vi "test_CCDAcquisitionSequenceSpectrum.vi"(0 "device selection":enum16{"monochromator", "CCD", "SCD"}(ring)=enum."CCD", 1 "Test should pass":bool=TRUE, 5 "set-up a connection":bool=TRUE, 7 "set 3 ROIs / set 1 ROI":bool=TRUE, 9 "tear down connection":bool=TRUE, 11 "error in":errorcluster, 12 "activate logger?":bool, 13 "Handler Name":string="example logger handler") -> (2 "ready":bool, 3 "log-file path":path, 4 "results-JSON string":string, 6 "xyData":dbl[][][][](array[numeric]), 8 "meta data":T1[][](array[typedef]), 15 "error out":errorcluster)   [LabVIEW 2023]
uses:
  Classes/CCD/CCDSpectralData.ctl
  Classes/CCD/XAxisConversionTypeEnum.ctl
  Classes/CCD/AcquisitionFormatEnum.ctl
  Classes/CCD/CCD.lvclass
  <vilib>/addons/_JKI Toolkits/Caraya/classes/Assert/Assert Not Error.vi
  <vilib>/addons/_JKI Toolkits/Caraya/classes/Test/Test.lvclass
  <vilib>/addons/_JKI Toolkits/Caraya/classes/Assert/Assert.lvclass
panel:
  # "Connector Pane"
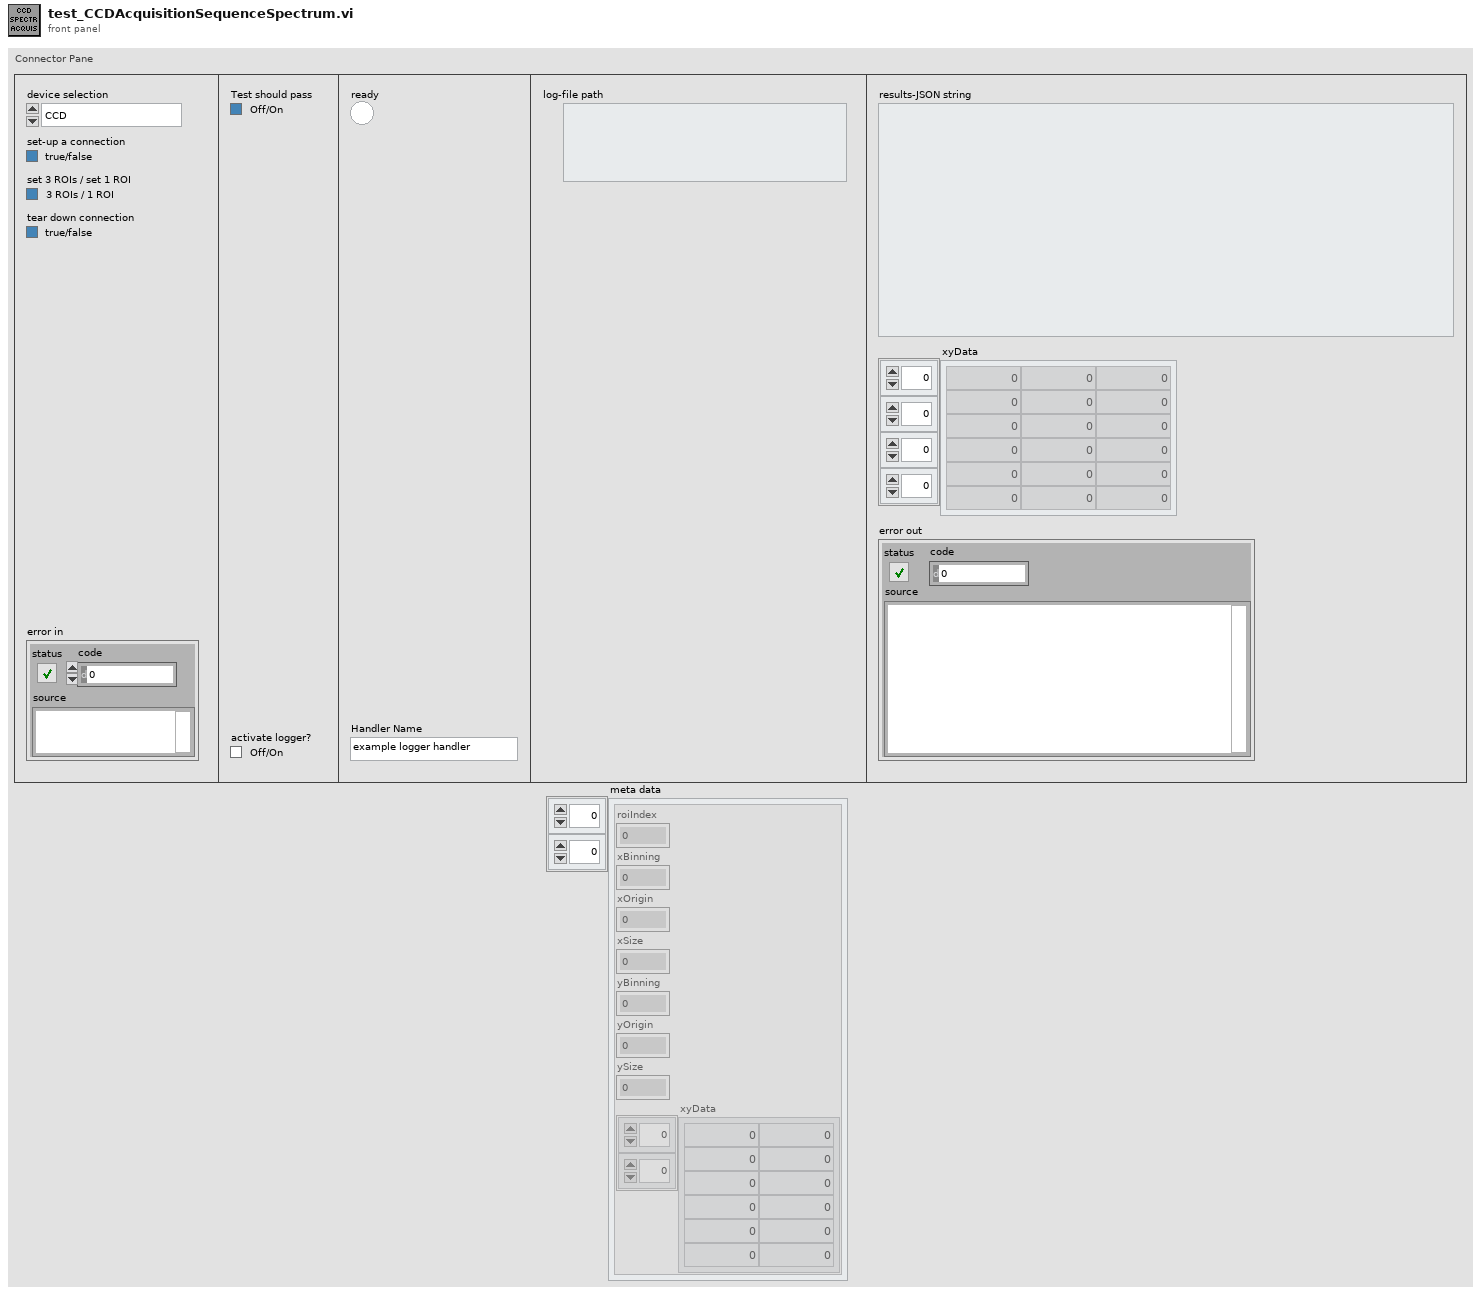
[diagram p1: front panel]
types:
  T1 = typedef "CCD.lvclass/CCDSpectralData.ctl" = cluster{"roiIndex":i32, "xBinning":i32, "xOrigin":i32, "xSize":i32, "yBinning":i32, "yOrigin":i32, "ySize":i32, "xyData":dbl[][]}
  T2 = typedef "CCD.lvclass/AcquisitionFormatEnum.ctl" = enum16{"Spectra", "Image", "Crop", "Fast Kinetics"}
  T3 = typedef "CCD.lvclass/XAxisConversionTypeEnum.ctl" = enum16{"None (default)", "CCD FIT parameters contained in the CCD firmware", "Mono Wavelength parameters contained in the icl_settings.ini file"}
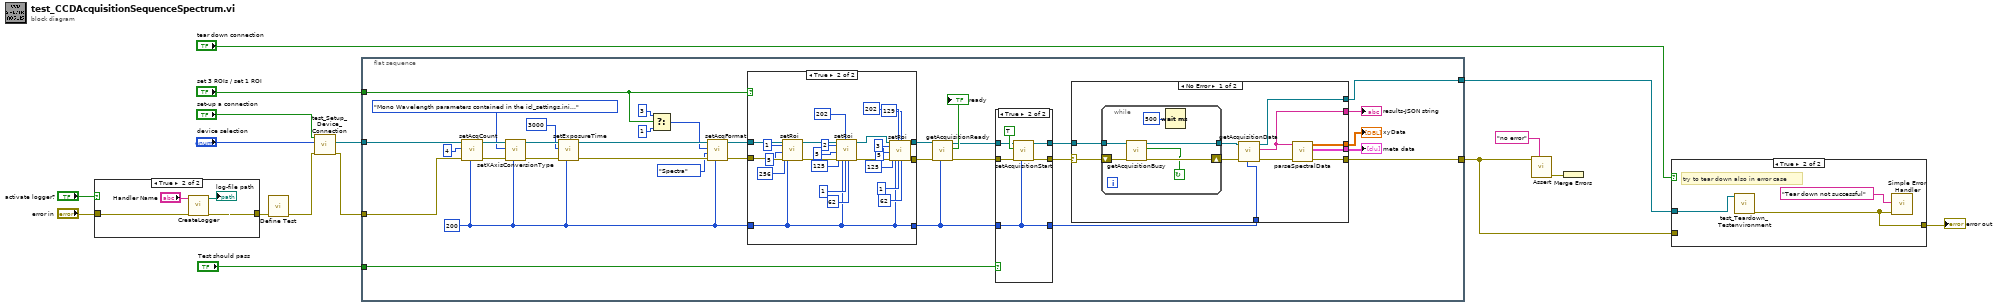
[diagram p0: block diagram]
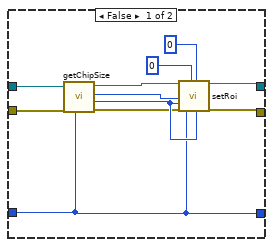
[diagram p2: hidden frame]
diagram:
  n1 = case shown="True" "activate logger?" {
    tunnel: [w17 w20] -> w2
    tunnel: "error in" -> [w17 w21]
    frame False {
    }
    frame True {
      n2 = call "CreateLogger.vi"("error in (no error)"=w21, "Handler Name"="Handler Name") -> ("error out"=w20:errorcluster, "log-file path"=→"log-file path":path)  [unwired: 8 in]
    }
  }
  n3 = call <vilib>:"Define Test.vi"("error in (no error)"=w2) -> ("error out"=w7:errorcluster)  [unwired: 9 in, 1 out]
  n4 = call "test_Setup_Device_Connection.vi"("error in (no error)"=w7, "device selection"="device selection", "set-up a connection"="set-up a connection") -> ("error out"=w8:errorcluster, "CCD.lvclass"=w9:refnum<class "CCD.lvclass">)  [unwired: 5 in, 2 out]
  n5 = flat-sequence {
    tunnel: w8 -> [w52]
    tunnel: w9 -> [w53]
    tunnel: [w40] -> w12
    tunnel: "Test should pass" -> [w54]
    tunnel: [w41] -> w11
    tunnel: "set 3 ROIs / set 1 ROI" -> [w33]
    frame #0 {
      w25 = 200 ("Delay between send and receive [ms]")
      n6 = call "setAcqCount.vi"("Delay between send and receive [ms]"=w25, "error in (no error)"=w52, "count"=4, "CCD in"=w53) -> ("error out"=w49:errorcluster, "CCD out"=w50:refnum<class "CCD.lvclass">)  [unwired: 4 in, 2 out]
      n7 = call "setXAxisConversionType.vi"("Delay between send and receive [ms]"=w25, "error in (no error)"=w49, "Enum"=XAxisConversionTypeEnum."Mono Wavelength parameters contained in the icl_settings.ini file", "CCD in"=w50) -> ("error out"=w47:errorcluster, "CCD out"=w46:refnum<class "CCD.lvclass">)  [unwired: 4 in, 2 out]
      n8 = call "setExposureTime.vi"("Delay between send and receive [ms]"=w25, "error in (no error)"=w47, "exposure time [ms] or [us]"=3000 ("exposure time [ms]"), "CCD in"=w46) -> ("error out"=w43:errorcluster, "CCD out"=w44:refnum<class "CCD.lvclass">)  [unwired: 4 in, 2 out]
      n9 = Select(t=3 ("number of ROIs"), s=w33, f=1) -> (s? t:f=w30:i32)
      n10 = call "setAcqFormat.vi"("Delay between send and receive [ms]"=w25, "error in (no error)"=w43, "acquisition format"=AcquisitionFormatEnum."Spectra", "number of ROIs"=w30, "CCD in"=w44) -> ("error out"=w36:errorcluster, "CCD out"=w37:refnum<class "CCD.lvclass">)  [unwired: 3 in, 2 out]
      n11 = case shown="True" w33 {
        tunnel: w37 -> [w57 w90]
        tunnel: w36 -> [w58 w89]
        tunnel: w25 -> [w59 w68]
        tunnel: [w59 w68] -> _
        tunnel: [w56 w67] -> w35
        tunnel: [w55 w66] -> w34
        frame False {
          n12 = call-dynamic "getChipSize.vi"("Delay between send and receive [ms]"=w59, "error in (no error)"=w58, "CCD in"=w57) -> ("error out"=w63:errorcluster, "chip size, y"=w65:i32, "chip size, x"=w64:i32, "CCD out"=w62:refnum<class "CCD.lvclass">)  [unwired: 5 in]
          n13 = call "setRoi.vi"("CCD in"=w62, "xSize"=w64, "ySize"=w65, "error in (no error)"=w63, "Delay between send and receive [ms]"=w59, "xOrigin"=0, "yOrigin"=0, "yBin"=w65) -> ("CCD out"=w56:refnum<class "CCD.lvclass">, "error out"=w55:errorcluster)  [unwired: 8 in, 2 out]
        }
        frame True {
          n14 = call "setRoi.vi"("CCD in"=w90, "ROI-index"=1, "xSize"=5, "ySize"=256, "error in (no error)"=w89, "Delay between send and receive [ms]"=w68) -> ("CCD out"=w88:refnum<class "CCD.lvclass">, "error out"=w87:errorcluster)  [unwired: 10 in, 2 out]
          n15 = call "setRoi.vi"("CCD in"=w88, "ROI-index"=2, "xSize"=5, "ySize"=125, "error in (no error)"=w87, "Delay between send and receive [ms]"=w68, "xOrigin"=202, "xBin"=1, "yBin"=62) -> ("CCD out"=w73:refnum<class "CCD.lvclass">, "error out"=w72:errorcluster)  [unwired: 7 in, 2 out]
          n16 = call "setRoi.vi"("CCD in"=w73, "ROI-index"=3, "xSize"=5, "ySize"=125, "error in (no error)"=w72, "Delay between send and receive [ms]"=w68, "xOrigin"=202, "xBin"=1, "yOrigin"=129, "yBin"=62) -> ("CCD out"=w67:refnum<class "CCD.lvclass">, "error out"=w66:errorcluster)  [unwired: 6 in, 2 out]
        }
      }
      n17 = call "getAcquisitionReady.vi"("Delay between send and receive [ms]"=w25, "error in (no error)"=w34, "CCD in"=w35) -> ("error out"=w29:errorcluster, "ready"=→"ready":bool, "CCD out"=w26:refnum<class "CCD.lvclass">)  [unwired: 6 in]
      n18 = case shown="True" w54 {
        tunnel: w26 -> [w110 w116]
        tunnel: w29 -> [w111 w115]
        tunnel: [w110 w113] -> w28
        tunnel: [w111 w114] -> w27
        tunnel: [w112 w117] -> w24
        tunnel: w25 -> [w112 w117]
        frame False {
        }
        frame True {
          n19 = call "setAcquisitionStart.vi"("Delay between send and receive [ms]"=w117, "error in (no error)"=w115, "openShutter"=TRUE, "CCD in"=w116) -> ("error out"=w114:errorcluster, "CCD out"=w113:refnum<class "CCD.lvclass">)  [unwired: 4 in, 2 out]
        }
      }
      n20 = case shown="No Error" w27 {
        selector: w27 -> [w97 w108]
        tunnel: w28 -> [w101 w109]
        tunnel: [w96 w109] -> w41
        tunnel: [w94 w108] -> w40
        tunnel: [w93 _] -> w39
        tunnel: w24 -> [w98 _]
        tunnel: [w91 _] -> w23
        tunnel: [w92 _] -> w22
        frame No Error {
          n21 = while {
            tunnel: w101 -> [w107]
            tunnel: [w106] -> w100
            shift-right: [w104] -> w99
            shift-left: w97 -> [w103]
            stop <- w102 continue-if-true
            n22 = call "getAcquisitionBusy.vi"("error in (no error)"=w103, "CCD in"=w107) -> ("error out"=w104:errorcluster, "isBusy"=w102:bool, "CCD out"=w106:refnum<class "CCD.lvclass">)  [unwired: 7 in]
            n23 = Wait (ms)(milliseconds to wait=u32 500) -> ()  [unwired: 1 out]
          }
          n24 = call "getAcquisitionData.vi"("Delay between send and receive [ms]"=w98, "error in (no error)"=w99, "CCD in"=w100) -> ("error out"=w95:errorcluster, "results-JSON string"=w93:string, "CCD out"=w96:refnum<class "CCD.lvclass">)  [unwired: 6 in]
          n25 = call "parseSpectralData.vi"("error in (no error)"=w95, "results-JSON string"=w93) -> ("error out"=w94:errorcluster, "meta data"=w92:T1[][], "xyData"=w91:dbl[][][][])  [unwired: 7 in]
        }
        frame Error {
        }
      }
      "results-JSON string" <- w39
      "xyData" <- w23
      "meta data" <- w22
    }
  }
  n26 = call-poly <vilib>:"Assert.vi"("Label"="no error" ("Label (VI Title)"), "Not Error?"=w12) -> ("error out"=w14:errorcluster)  [unwired: 8 in, 1 out]
  n27 = Merge Errors(w14) -> ()  [unwired: 1 out]
  n28 = case shown="True" "tear down connection" {
    tunnel: w11 -> [_ w121]
    tunnel: [w119 w120] -> w10
    tunnel: w12 -> [w119 _]
    frame False {
    }
    frame True {
      # "try to tear down also in error case"
      n29 = call "test_Teardown_Testenvironment.vi"("GenericDevice.lvclass"=w121) -> ("error out"=w120:errorcluster)  [unwired: 9 in, 1 out]
      n30 = call <vilib>:"Simple Error Handler.vi"("error source (\" \")"="Tear down not successful" ("error source (\" \")"), "error in (no error)"=w120) -> ()  [unwired: 3 in, 5 out]
    }
  }
  "error out" <- w10
